vi "sendvalue.vi"(6 "addr/port":cluster{"address":string, "port":i32}, 8 "error in (no error)":errorcluster, 10 "numerical value":dbl format="%#_13g", 11 "command string":string) -> (0 "error out":errorcluster, 2 "bytes written":i32, 3 "connection ID out":refnum<k5>)   [LabVIEW 2015]
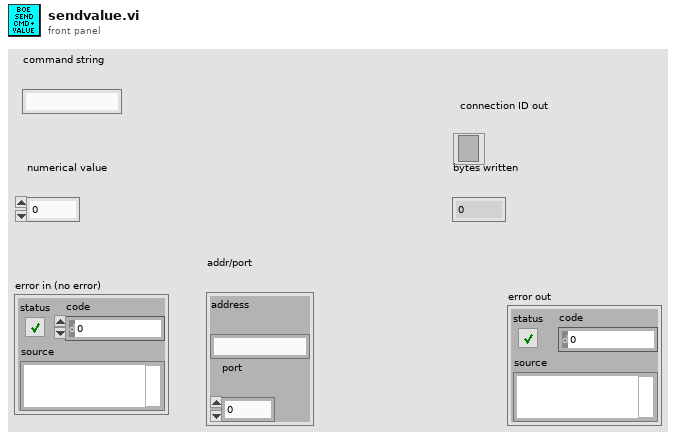
[diagram p1: front panel]
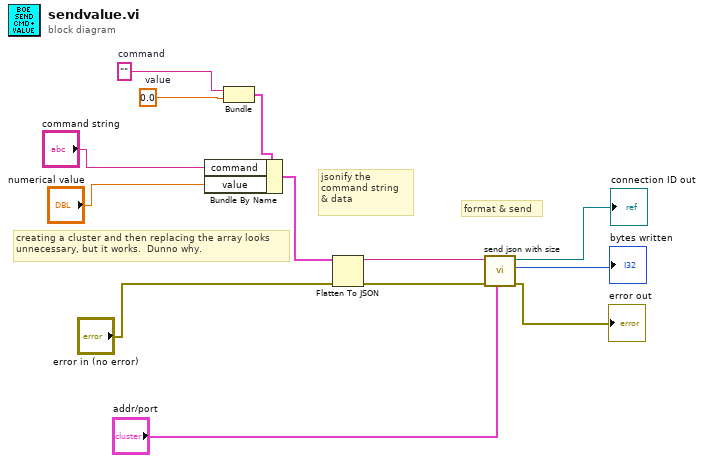
[diagram p0: block diagram]
diagram:
  w11 = 0.0  # value
  w12 = ""  # command
  # "format & send"
  # "creating a cluster and then replacing the array looks\nunnecessary, but it works.  Dunno why."
  # "jsonify the \ncommand string \n& data"
  n1 = Bundle("command"=w12, "value"=w11) -> (w10:cluster{"command":string, "value":dbl})  [unwired: 1 in]
  n2 = Bundle By Name(cluster=w10, "command"="command string", "value"="numerical value") -> (w7:cluster{"command":string, "value":dbl})
  n3 = Flatten To JSON(anything=w7, error in (no error)="error in (no error)") -> (JSON string=w6:string, 11:w5:errorcluster)  [unwired: 1 in]
  n4 = call "send json with size.vi"("addr/port"="addr/port", "error in"=w5, "json string"=w6) -> ("error out"=→"error out":errorcluster, "bytes written"=→"bytes written":i32, "connection ID out"=→"connection ID out":refnum<k5>)  [unwired: 6 in]
